vi "AutoCAD busy NET.vi"(6 "error in (no error)":errorcluster, 7 "Application 2":refnum<k24>) -> (2 "error out":errorcluster, 3 "IsQuiescent":bool)   [LabVIEW 2010]
uses:
  Autodesk.AutoCAD.Interop
panel:
  out "Numeric":i32
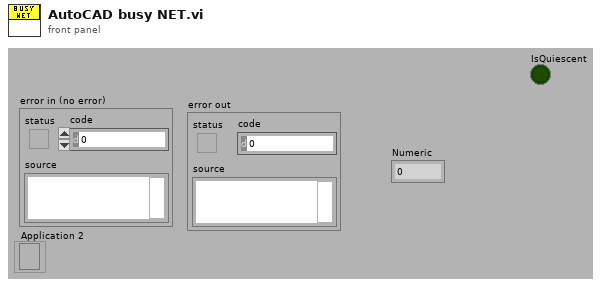
[diagram p1: front panel]
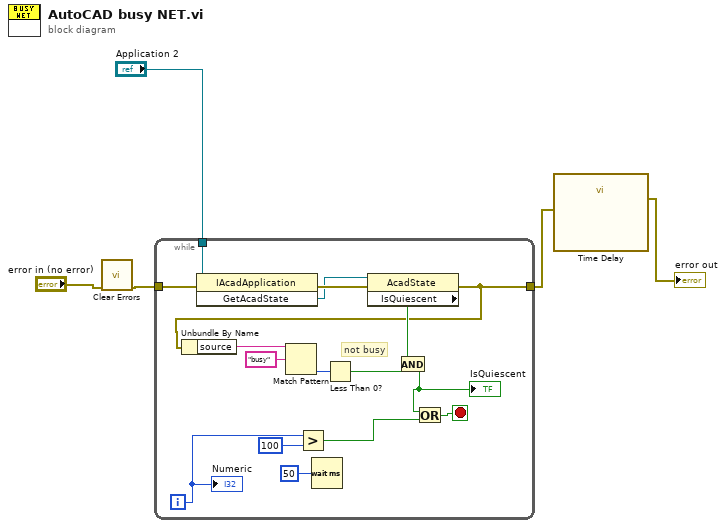
[diagram p0: block diagram]
diagram:
  n1 = call <vilib>:"Clear Errors.vi"("error in (no error)"="error in (no error)") -> ("error out"=w4:errorcluster)  [unwired: 6 in]
  n2 = while {
    tunnel: "Application 2" -> [w21]
    tunnel: w4 -> [w13]
    tunnel: [w12] -> w3
    i -> [w16]
    stop <- w15 stop-if-true
    # "not busy"
    n3 = invoke class="IAcadApplication" method="GetAcadState"(reference=w21, error in=w13) -> (error out=w20:errorcluster, "GetAcadState"=w6:refnum<k24>)  [unwired: 1 in, 1 out]
    n4 = Greater?(x=w16, y=100) -> (0:w18:bool)
    n5 = Wait (ms)(milliseconds to wait=u32 50) -> ()  [unwired: 1 out]
    n6 = property class="AcadState"(reference=w6, error in=w20) -> (error out=w12:errorcluster, "IsQuiescent"=w14:bool)  [unwired: 1 out]
    n7 = Unbundle By Name(w12) -> ("source"=w11:string)
    n8 = Match Pattern(string=w11, regular expression="busy") -> (offset past match=w9:i32)  [unwired: 1 in, 3 out]
    n9 = Less Than 0?(x=w9) -> (x < 0?=w8:bool)
    n10 = And(x=w14, y=w8) -> (x .and. y?=w7:bool)
    "IsQuiescent" <- w7
    n11 = Or(x=w7, y=w18) -> (x .or. y?=w15:bool)
    "Numeric" <- w16
  }
  n12 = call "Time Delay"("error in (no error)"=w3) -> ("error out"=→"error out":errorcluster)  [unwired: 10 in]
